vi "MiniCanSat 2018.vi"() -> ()   [LabVIEW 2015]
uses:
  <vilib>/Instr/_visa.llb/VISA Configure Serial Port (Instr).vi
panel:
  out "Ground Speed":dbl(knob) scale=0.0..120.0
  out "Dial":dbl(knob) scale=0.0..360.0
  out "XY Graph":cluster{dbl[], dbl[]}(graph)
  in  "file path":path
  out "Speed":dbl
  out "Longitude":string
  out "Latitude":string
  out "Direction":string
  in  "stop":bool
  in  "VISA resource name":refnum<visa-resource-name>
  # "Ground Station : Mini CANSAT 2018"
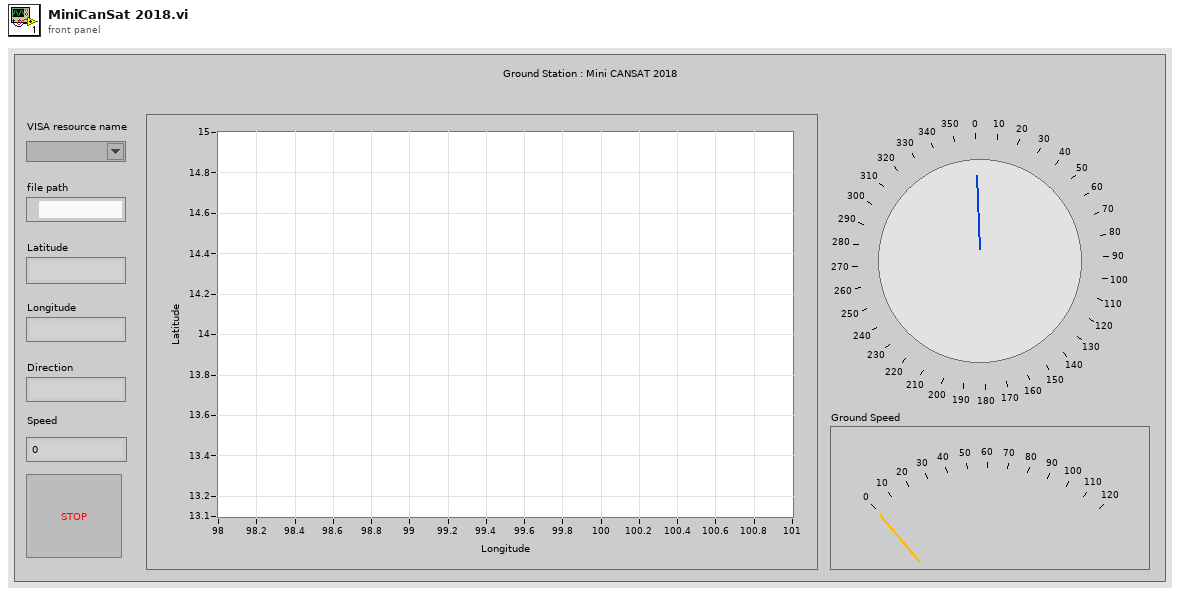
[diagram p1: front panel]
types:
  T1 = enum16{"open", "replace", "create", "open or create", "replace or create", "replace or create with confirmation"}
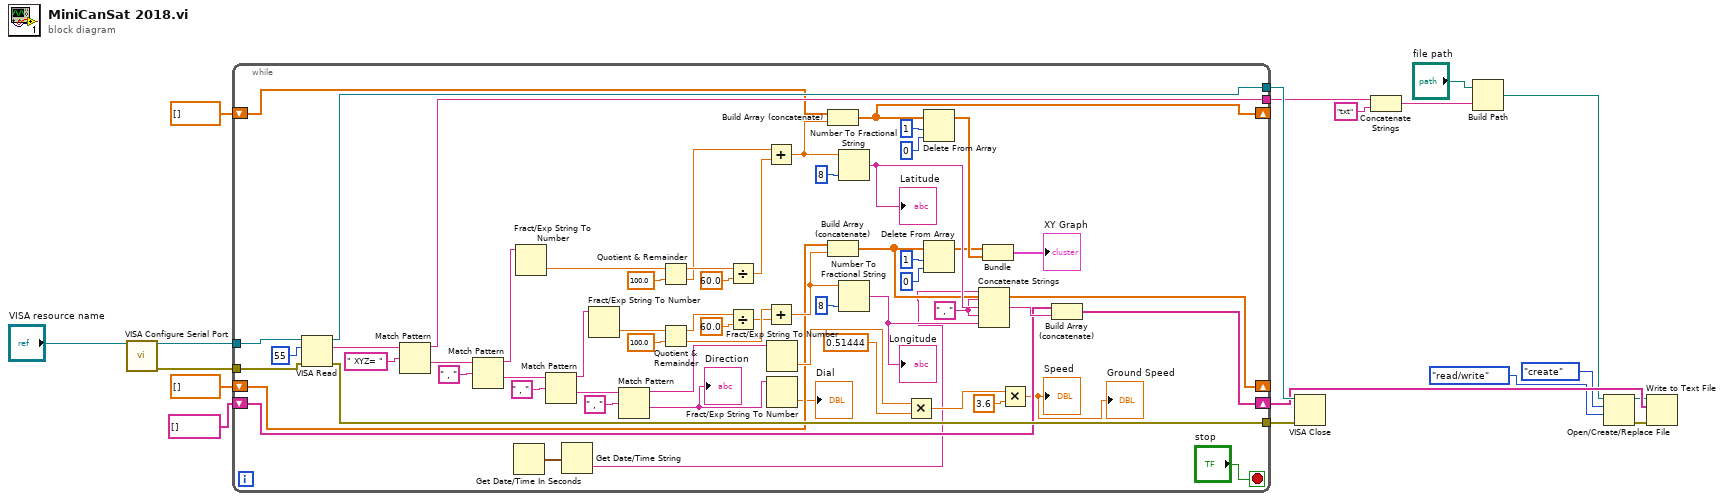
[diagram p0: block diagram]
diagram:
  n1 = call-poly "VISA Configure Serial Port"("VISA resource name"="VISA resource name") -> ("VISA resource name out"=w17:refnum<visa-resource-name>, "error out"=w16:errorcluster)  [unwired: 13 in]
  n2 = while {
    tunnel: w17 -> [w78]
    tunnel: w16 -> [w77]
    tunnel: [w75] -> w15
    tunnel: [w74] -> w14
    shift-right: [w39] -> w12
    shift-left: string[] [] -> [w40]
    tunnel: [w38] -> w5
    shift-right: [w27] -> _
    shift-left: dbl[] [] -> [w36]
    shift-right: [w32] -> _
    shift-left: dbl[] [] -> [w34]
    stop <- "stop" stop-if-true
    w20 = " , " ("string")
    n3 = VISA Read(VISA resource name=w78, byte count=u32 55, error in (no error)=w77) -> (VISA resource name out=w75:refnum<visa-resource-name>, read buffer=w71:string, error out=w74:errorcluster)  [unwired: 1 out]
    n4 = Match Pattern(string=w71, regular expression=" XYZ= ") -> (before substring=w38:string, after substring=w69:string)  [unwired: 1 in, 2 out]
    n5 = Match Pattern(string=w69, regular expression=" , ") -> (before substring=w64:string, after substring=w66:string)  [unwired: 1 in, 2 out]
    n6 = Get Date/Time In Seconds() -> (seconds since 1Jan1904=w21:timestamp)
    n7 = Fract/Exp String To Number(string=w64) -> (number=w62:dbl)  [unwired: 3 in, 1 out]
    n8 = Match Pattern(string=w66, regular expression=" , ") -> (before substring=w63:string, after substring=w65:string)  [unwired: 1 in, 2 out]
    n9 = Get Date/Time String(seconds (now)=w21) -> (time string=w19:string)  [unwired: 2 in, 1 out]
    n10 = Fract/Exp String To Number(string=w63) -> (number=w59:dbl)  [unwired: 3 in, 1 out]
    n11 = Match Pattern(string=w65, regular expression=" , ") -> (before substring=w58:string, after substring=w24:string)  [unwired: 1 in, 2 out]
    "Direction" <- w24
    n12 = Quotient & Remainder(x=w62, y=100.0) -> (x-y*floor(x/y)=w50:dbl, floor(x/y)=w46:dbl)
    n13 = Quotient & Remainder(x=w59, y=100.0) -> (x-y*floor(x/y)=w48:dbl, floor(x/y)=w45:dbl)
    n14 = Divide(x=w50, y=60.0) -> (x/y=w47:dbl)
    n15 = Divide(x=w48, y=60.0) -> (x/y=w44:dbl)
    n16 = Add(x=w46, y=w47) -> (x+y=w35:dbl)
    n17 = Add(x=w45, y=w44) -> (x+y=w37:dbl)
    n18 = Fract/Exp String To Number(string=w58) -> (number=w57:dbl)  [unwired: 3 in, 1 out]
    n19 = Fract/Exp String To Number(string=w24) -> (number=→"Dial":dbl)  [unwired: 3 in, 1 out]
    n20 = Build Array (concatenate)(w34, w35) -> (w32:dbl[])
    n21 = Build Array (concatenate)(w36, w37) -> (w27:dbl[])
    n22 = Number To Fractional String(number=w35, precision (6)=i16 8) -> (F-format string=w43:string)  [unwired: 2 in]
    "Latitude" <- w43
    n23 = Number To Fractional String(number=w37, precision (6)=i16 8) -> (F-format string=w42:string)  [unwired: 2 in]
    "Longitude" <- w42
    n24 = Multiply(x=w57, y=0.51444) -> (x*y=w55:dbl)
    n25 = Delete From Array(array=w32, length=1, index=0) -> (array with subset deleted=w26:dbl[])  [unwired: 1 out]
    n26 = Delete From Array(array=w27, length=1, index=0) -> (array with subset deleted=w25:dbl[])  [unwired: 1 out]
    n27 = Concatenate Strings(w19, w20, w43, w20, w42) -> (w41:string)
    n28 = Bundle(w25, w26) -> (→"XY Graph":cluster{dbl[], dbl[]})  [unwired: 1 in]
    n29 = Multiply(x=w55, y=3.6) -> (x*y=→"Speed" →"Ground Speed":dbl)
    n30 = Build Array (concatenate)(w40, w41) -> (w39:string[])
  }
  n31 = VISA Close(VISA resource name=w15, error in (no error)=w14) -> ()  [unwired: 1 out]
  n32 = Concatenate Strings(w5, "txt" ("string")) -> (w4:string)
  n33 = Build Path(base path="file path", name or relative path=w4) -> (appended path=w7:path)
  n34 = Open/Create/Replace File(file path (use dialog)=w7, operation (0:open)=T1."create", access (0:read/write)=enum16{"read/write", "read-only", "write-only"}."read/write") -> (refnum out=w11:refnum<file>, error out=w10:errorcluster)  [unwired: 3 in, 1 out]
  n35 = Write to Text File(file (use dialog)=w11, text=w12, error in=w10) -> ()  [unwired: 1 in, 3 out]
